vi "AnalyseClassFile.vi"(11 "File Path":path) -> (2 "IsInterface":bool, 3 "ParentLibraries":path[](array[path]))   [LabVIEW 2020, in "DependencyChecker.lvlib"]
uses:
  DependencyChecker.lvlib
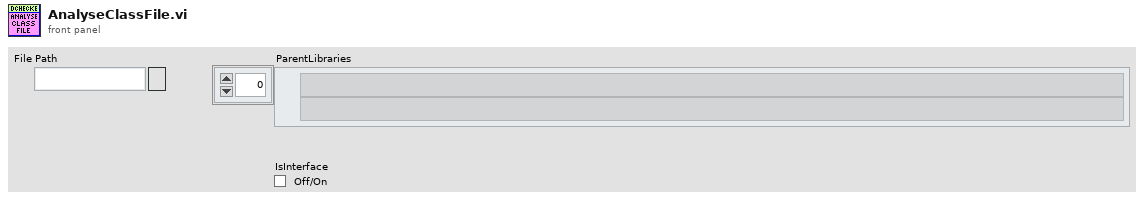
[diagram p1: front panel]
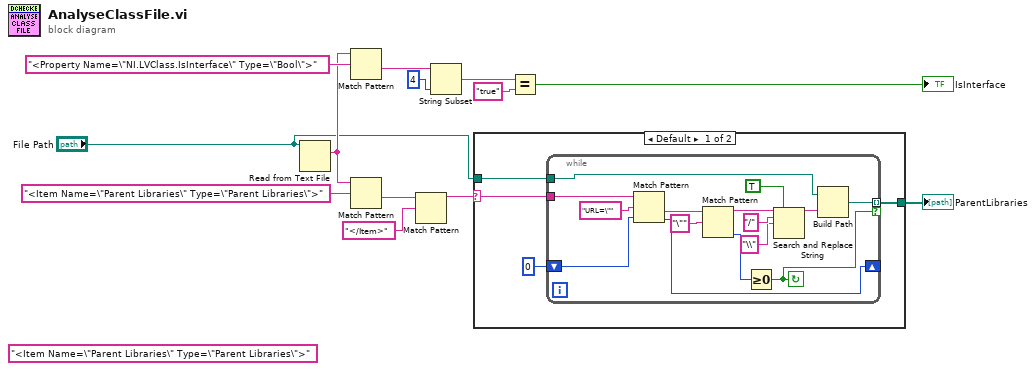
[diagram p0: block diagram]
diagram:
  (unwired) "<Item Name=\"Parent Libraries\" Type=\"Parent Libraries\">" ("regular expression")
  n1 = Read from Text File(file (use dialog)="File Path") -> (text=w3:string)  [unwired: 3 in, 3 out]
  n2 = Match Pattern(string=w3, regular expression="<Property Name=\"NI.LVClass.IsInterface\" Type=\"Bool\">") -> (after substring=w12:string)  [unwired: 1 in, 3 out]
  n3 = Match Pattern(string=w3, regular expression="<Item Name=\"Parent Libraries\" Type=\"Parent Libraries\">") -> (after substring=w7:string)  [unwired: 1 in, 3 out]
  n4 = Match Pattern(string=w7, regular expression="</Item>") -> (before substring=w4:string)  [unwired: 1 in, 3 out]
  n5 = String Subset(string=w12, length (rest)=4 ("length (rest)")) -> (substring=w10:string)  [unwired: 1 in]
  n6 = case shown="Default" w4 {
    selector: w4 -> [w17 _]
    tunnel: "File Path" -> [w16 _]
    tunnel: [w15 _] -> w2
    frame Default {
      n7 = while {
        tunnel: w17 -> [w32]
        tunnel: w16 -> [w27]
        tunnel: [w26] -> w15 mode=indexing if=w25
        shift-right: [w23] -> _
        shift-left: 0 ("offset past match") -> [w24]
        stop <- w25 continue-if-true
        n8 = Match Pattern(string=w32, regular expression="URL=\"", offset (0)=w24) -> (after substring=w30:string, offset past match=w23:i32)  [unwired: 2 out]
        n9 = Match Pattern(string=w30, regular expression="\"") -> (before substring=w22:string, offset past match=w28:i32)  [unwired: 1 in, 2 out]
        n10 = Greater Or Equal To 0?(x=w28) -> (x >= 0?=w25:bool)
        n11 = Search and Replace String(replace all?=TRUE ("replace all? (F)"), input string=w22, search string="/", replace string="\\" ("replace string (\"\")")) -> (result string=w18:string)  [unwired: 4 in, 3 out]
        n12 = Build Path(base path=w27, name or relative path=w18) -> (appended path=w26:path)
      }
    }
    frame "" {
    }
  }
  "ParentLibraries" <- w2
  n13 = Equal?(x=w10, y="true") -> (x = y?=→"IsInterface":bool)
